vi "Var_Locales.vi"() -> ()   [LabVIEW 2021]
panel:
  in  "TIEMPO C":u32
  in  "TIEMPO P":u32
  out "W C":dbl(graph)
  out "W P":dbl(graph)
  out "CONTADOR C":i32
  in  "stop":bool
  out "CONTADOR P":i32
  # "MENDOZA MEZA MANUEL EVERARDO"
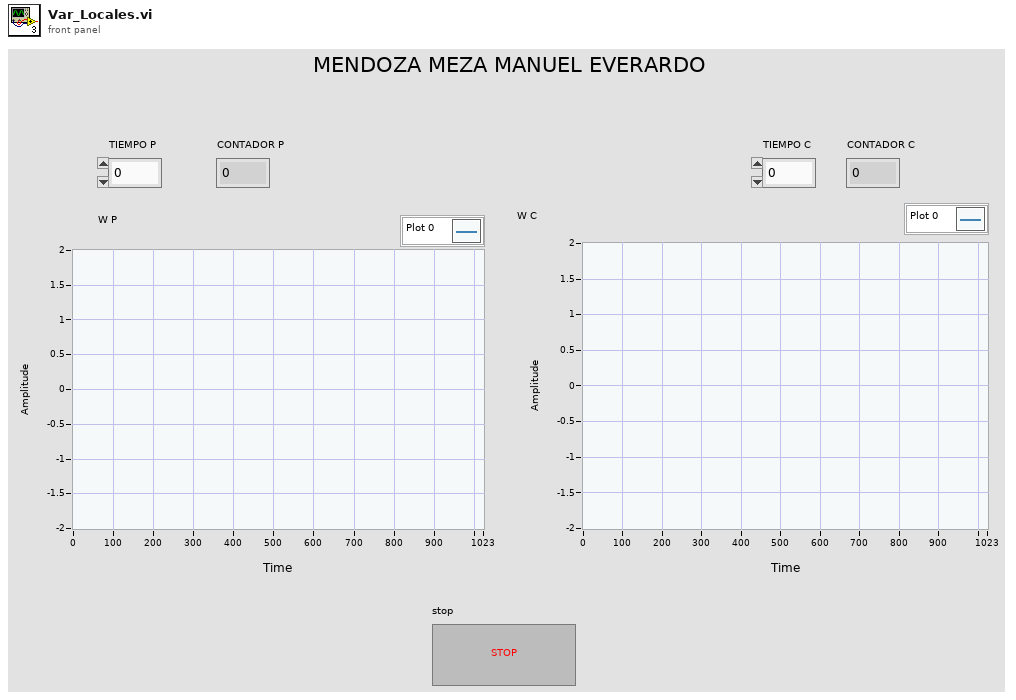
[diagram p1: front panel]
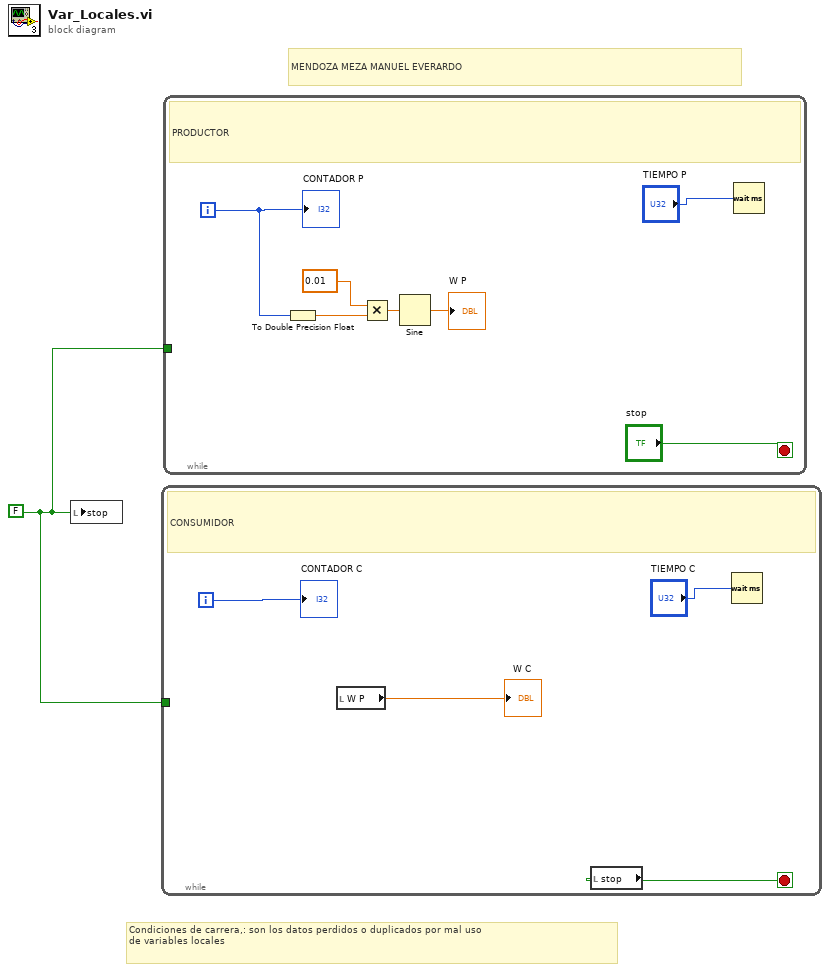
[diagram p0: block diagram]
diagram:
  w1 = FALSE ("stop")
  # "Condiciones de carrera,: son los datos perdidos o duplicados por mal uso\nde variables locales"
  # "MENDOZA MEZA MANUEL EVERARDO"
  n1 = local write "stop"(w1) -> ()
  n2 = while {
    tunnel: w1 -> [_]
    i -> [w5]
    stop <- w4 stop-if-true
    # "CONSUMIDOR"
    n3 = local read "W P"() -> (→"W C":dbl)
    n4 = local read "stop"() -> (w4:bool)
    n5 = Wait (ms)(milliseconds to wait="TIEMPO C") -> ()  [unwired: 1 out]
    "CONTADOR C" <- w5
  }
  n6 = while {
    tunnel: w1 -> [_]
    i -> [w10]
    stop <- "stop" stop-if-true
    # "PRODUCTOR"
    n7 = To Double Precision Float(number=w10) -> (double precision float=w9:dbl)
    n8 = Multiply(x=0.01, y=w9) -> (x*y=w8:dbl)
    n9 = Sine(x=w8) -> (sin(x)=→"W P":dbl)
    n10 = Wait (ms)(milliseconds to wait="TIEMPO P") -> ()  [unwired: 1 out]
    "CONTADOR P" <- w10
  }
